vi "generate-analog-out-multiple-channels.vi"(11 "error in":errorcluster) -> (15 "error out":errorcluster)   [LabVIEW 2020]
uses:
  <vilib>/Utility/error.llb/DialogType.ctl
  <vilib>/DAQmx/write.llb/DAQmx Write (Analog 1D Wfm NChan NSamp).vi
  <vilib>/Utility/file.llb/Read Delimited Spreadsheet (string).vi
  <vilib>/DAQmx/create/channels.llb/DAQmx Create Channel (AO-Voltage-Basic).vi
  <vilib>/DAQmx/configure/timing.llb/DAQmx Timing (Use Waveform).vi
  <vilib>/DAQmx/miscellaneous.llb/DAQmx Fill In Error Info.vi
panel:
  out "Waveform Chart 4":waveform(dbl)(graph)
  out "Waveform Chart 3":waveform(dbl)(graph)
  out "number of samples written per channel":u32
  out "all rows of data":string[][](array[string])
  out "subarray":dbl[](array[numeric])
  in  "Array":dbl[][](array[numeric])
  out "Waveform Chart 2":waveform(dbl)(graph)
  out "Waveform Chart 1":waveform(dbl)(graph)
  out "Waveform Chart All":waveform(dbl)[](graph)
  in  "Delta T":dbl=0.0005
  in  "stop":bool
  in  "Physical Channel CH0":tag="DAQ1/ao0"
  in  "EMG Data File":path=path "C:/data/four-columns-of-data-by100.csv"
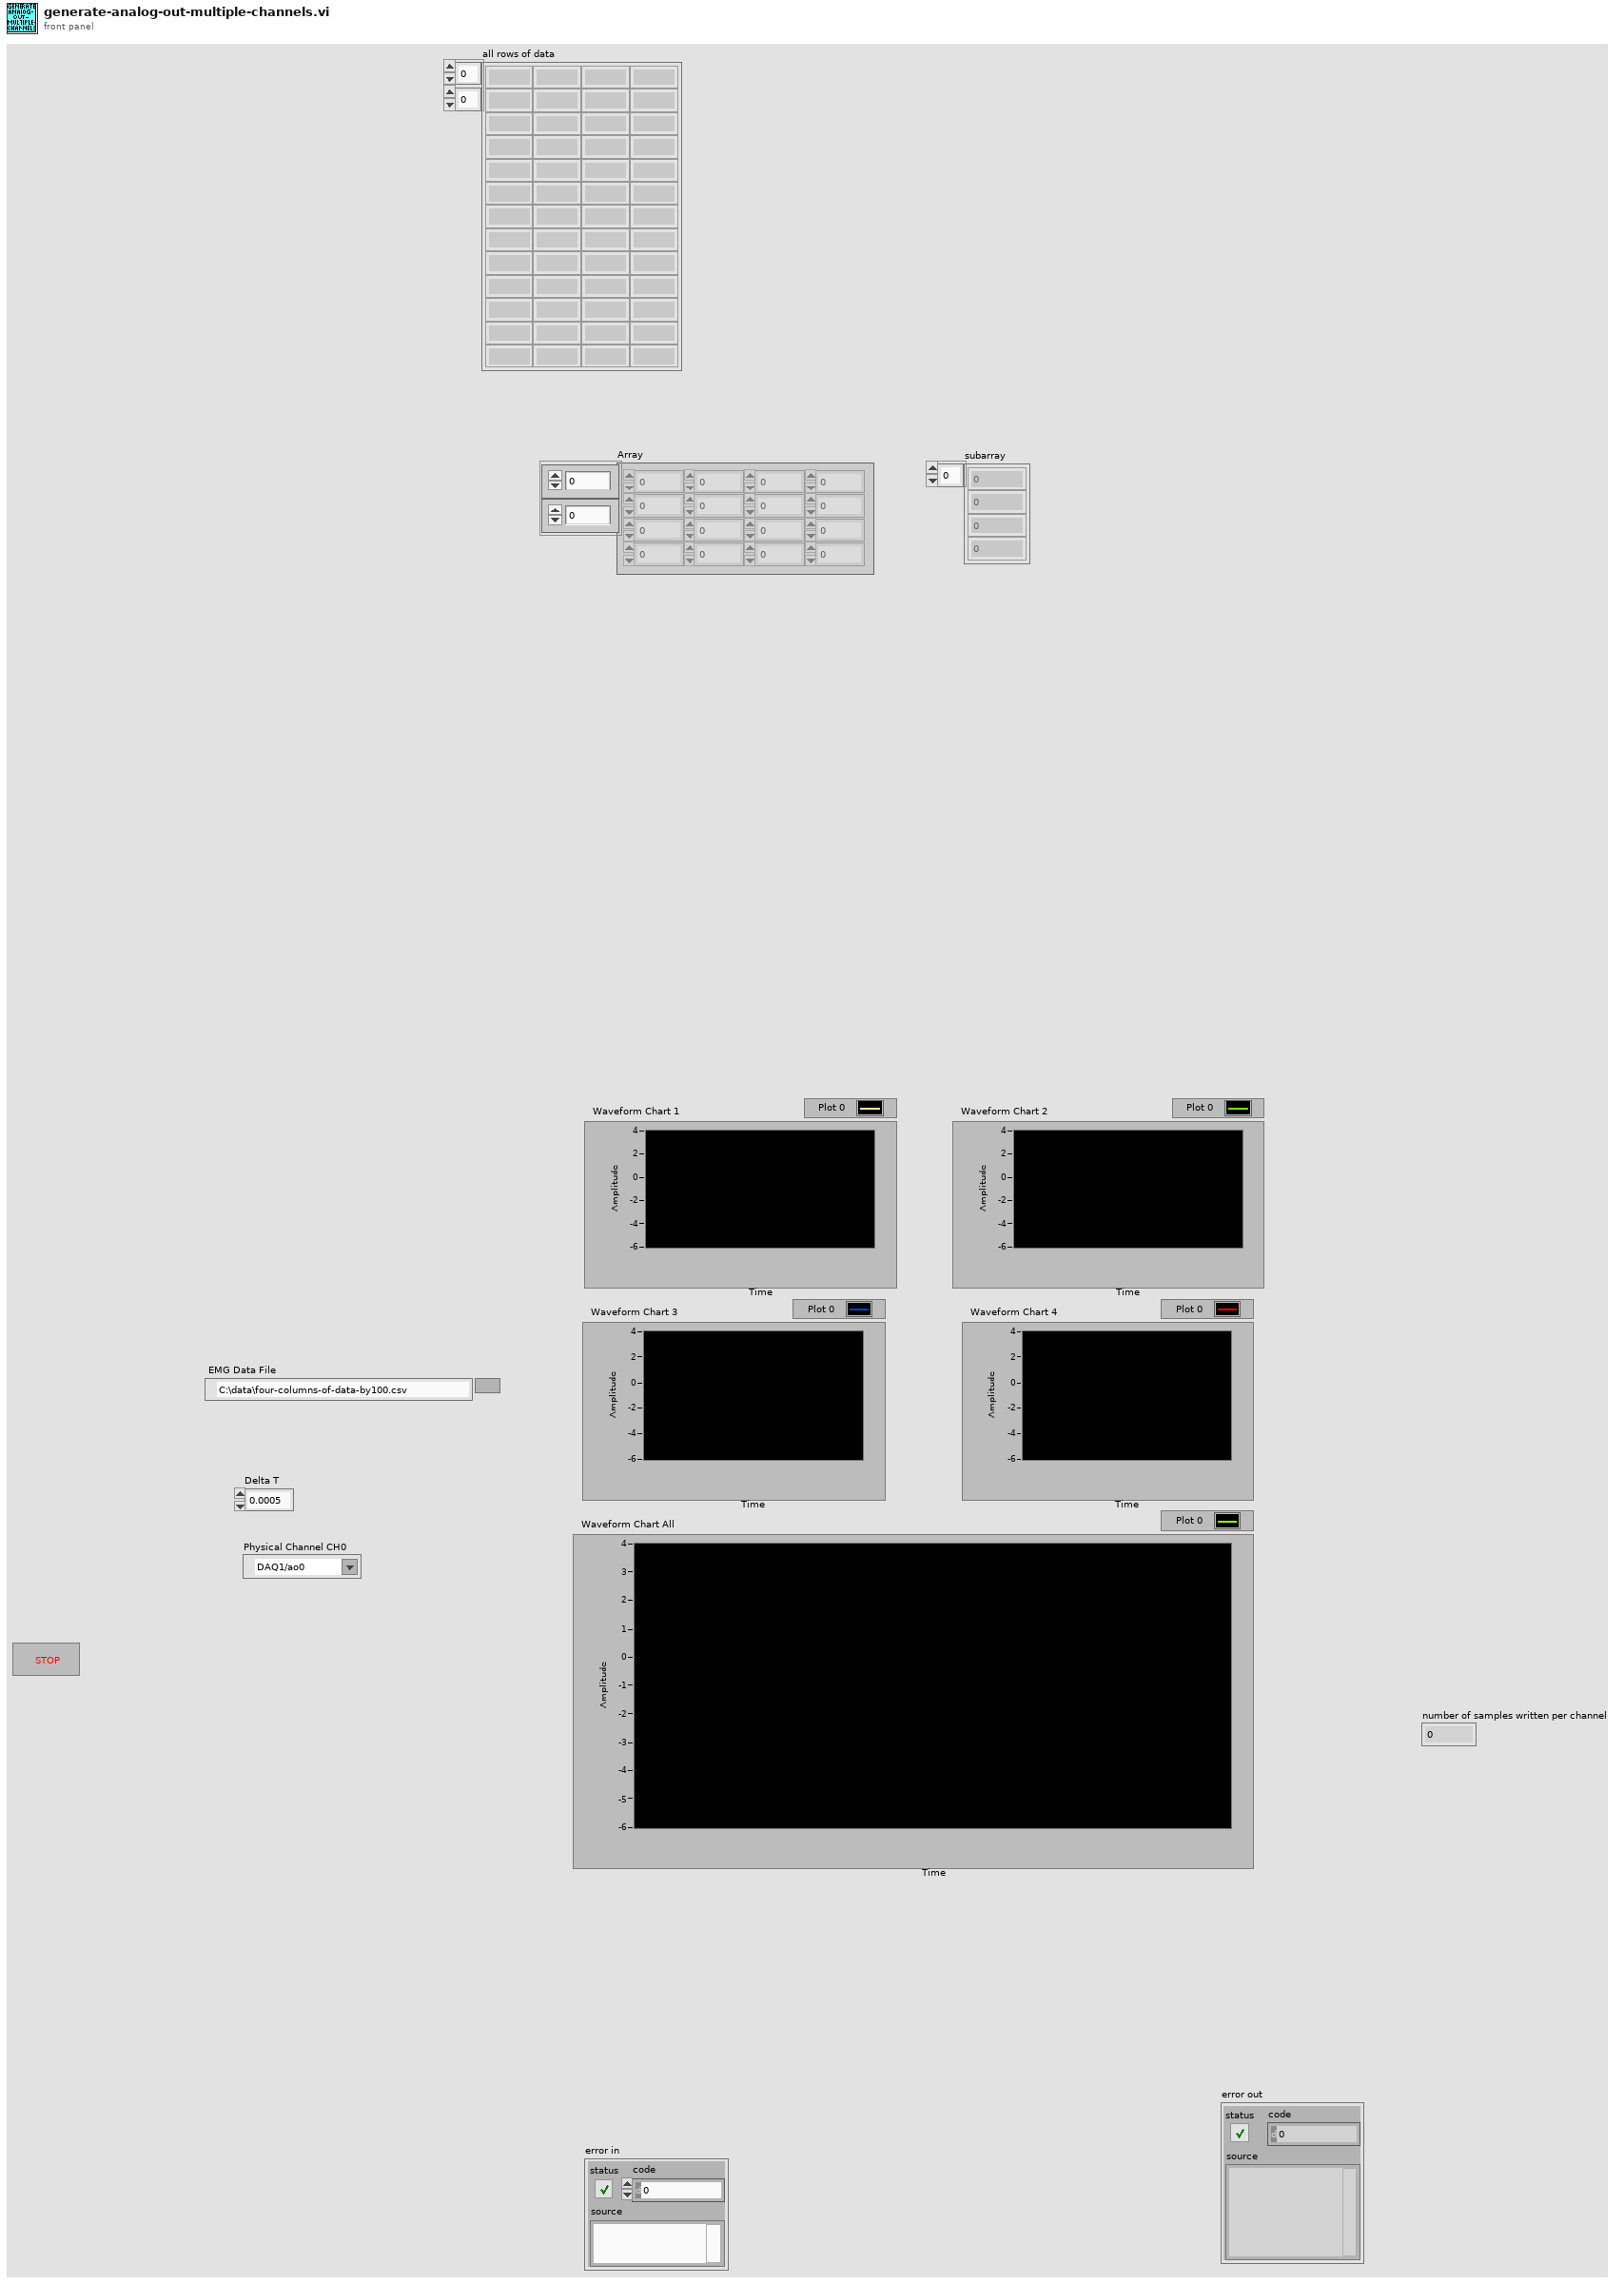
[diagram p1: front panel]
types:
  T1 = typedef "DialogType.ctl" = u16
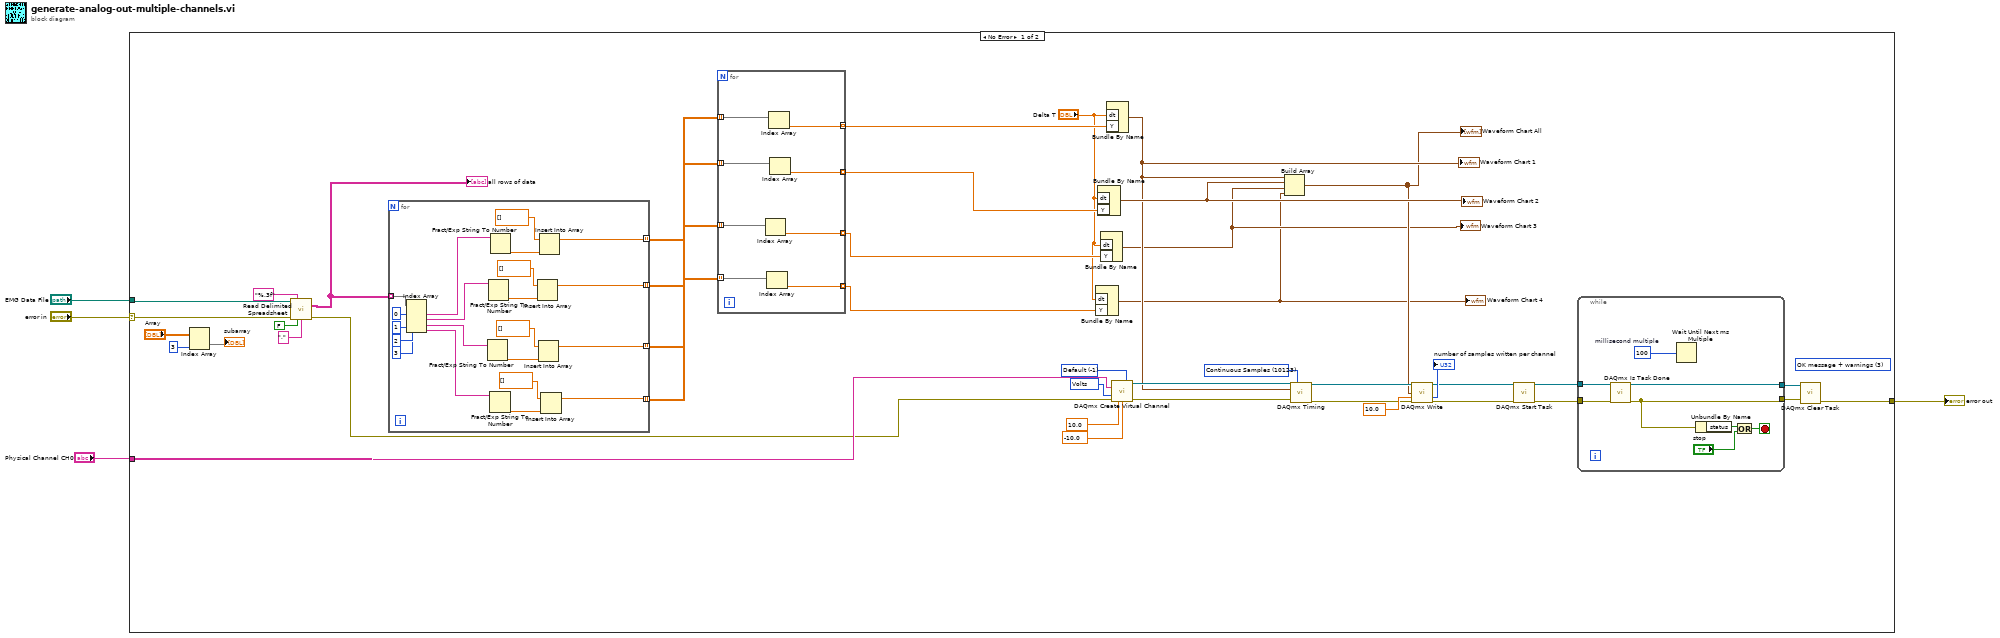
[diagram p0: block diagram]
diagram:
  n1 = case shown="No Error" "error in" {
    selector: "error in" -> [w25 w85]
    tunnel: [w7 w85] -> w3
    tunnel: "EMG Data File" -> [w29 _]
    tunnel: "Physical Channel CH0" -> [w35 _]
    frame No Error {
      w36 = 10348 items=["Volts"=10348, "From Custom Scale"=10065] ("units")
      w37 = -1 items=["Default"=-1, "RSE"=10083, "Differential"=10106, "Pseudodifferential"=12529] ("output terminal configuration")
      (unwired) T1 3 items=["no dialog", "OK message", "continue or stop message", "OK message + warnings", "continue/stop + warnings"] ("type of dialog (OK msg:1)")
      w47 = 10123 items=["Finite Samples"=10178, "Continuous Samples"=10123] ("sample mode")
      n2 = Index Array(array="Array", index (col)=3 ("disabled index (col)")) -> (element=→"subarray":dbl[])  [unwired: 1 in]
      n3 = call-poly <vilib>:"Read Delimited Spreadsheet.vi"("file path (dialog if empty)"=w29, "format (%s)"="%.3f" ("format (%.3f)"), "error in (no error)"=w25, "transpose? (F)"=FALSE, "delimiter (\\t)"="," ("delimiter (\\t)")) -> ("all rows"=w24:string[][], "error out"=w14:errorcluster)  [unwired: 5 in, 4 out]
      "all rows of data" <- w24
      n4 = for {
        tunnel: w24 -> [w76] mode=indexing
        tunnel: [w70] -> w23 mode=indexing
        tunnel: [w61] -> w21 mode=indexing
        tunnel: [w60] -> w19 mode=indexing
        tunnel: [w57] -> w18 mode=indexing
        n5 = Index Array(array=w76, index #1=0 ("index"), index #2=1 ("index"), index #3=2 ("index"), index #4=3 ("index")) -> (element #1=w68:string, element #2=w63:string, element #3=w62:string, element #4=w56:string)
        n6 = Fract/Exp String To Number(string=w62) -> (number=w65:dbl)  [unwired: 3 in, 1 out]
        n7 = Fract/Exp String To Number(string=w63) -> (number=w67:dbl)  [unwired: 3 in, 1 out]
        n8 = Fract/Exp String To Number(string=w56) -> (number=w59:dbl)  [unwired: 3 in, 1 out]
        n9 = Fract/Exp String To Number(string=w68) -> (number=w71:dbl)  [unwired: 3 in, 1 out]
        n10 = Insert Into Array(array=dbl[] [] ("Y"), new element=w67) -> (w61:dbl[])  [unwired: 1 in]
        n11 = Insert Into Array(array=dbl[] [], new element=w65) -> (w60:dbl[])  [unwired: 1 in]
        n12 = Insert Into Array(array=dbl[] [] ("Y"), new element=w71) -> (w70:dbl[])  [unwired: 1 in]
        n13 = Insert Into Array(array=dbl[] [], new element=w59) -> (w57:dbl[])  [unwired: 1 in]
      }
      n14 = for {
        tunnel: w23 -> [w55] mode=indexing
        tunnel: [w54] -> w22 mode=indexing
        tunnel: w21 -> [w53] mode=indexing
        tunnel: [w52] -> w20 mode=indexing
        tunnel: w19 -> [w51] mode=indexing
        tunnel: w18 -> [w50] mode=indexing
        tunnel: [w49] -> w10 mode=indexing
        tunnel: [w48] -> w8 mode=indexing
        n15 = Index Array(array=w51) -> (element=w49:dbl)  [unwired: 1 in]
        n16 = Index Array(array=w50) -> (element=w48:dbl)  [unwired: 1 in]
        n17 = Index Array(array=w55) -> (element=w54:dbl)  [unwired: 1 in]
        n18 = Index Array(array=w53) -> (element=w52:dbl)  [unwired: 1 in]
      }
      n19 = Bundle By Name("dt"="Delta T", "Y"=w8) -> (w5:waveform(dbl))  [unwired: 1 in]
      "Waveform Chart 4" <- w5
      n20 = Bundle By Name("dt"="Delta T", "Y"=w20) -> (w17:waveform(dbl))  [unwired: 1 in]
      "Waveform Chart 2" <- w17
      n21 = Bundle By Name("dt"="Delta T", "Y"=w10) -> (w6:waveform(dbl))  [unwired: 1 in]
      "Waveform Chart 3" <- w6
      n22 = Bundle By Name("dt"="Delta T", "Y"=w22) -> (w12:waveform(dbl))  [unwired: 1 in]
      "Waveform Chart 1" <- w12
      n23 = call-poly <vilib>:"DAQmx Create Virtual Channel.vi"("maximum value"=10.0 ("Maximum Value"), "minimum value"=-10.0 ("Minimum Value"), "output terminal configuration"=w37, "physical channels"=w35, "units"=w36, "error in"=w14) -> ("task out"=w34:refnum<k21>, "error out"=w33:errorcluster)  [unwired: 8 in]
      n24 = Build Array(w12, w17, w6, w5) -> (w11:waveform(dbl)[])
      "Waveform Chart All" <- w11
      n25 = call-poly <vilib>:"DAQmx Timing.vi"("task/channels in"=w34, "sample mode"=w47, "waveform"=w12, "error in"=w33) -> ("task out"=w16:refnum<k21>, "error out"=w40:errorcluster)  [unwired: 10 in]
      n26 = call-poly <vilib>:"DAQmx Write.vi"("task/channels in"=w16, "data"=w11, "timeout"=10.0 ("Wirite Timeout"), "error in"=w40) -> ("task out"=w13:refnum<k21>, "number of samples written per channel"=→"number of samples written per channel":u32, "error out"=w46:errorcluster)  [unwired: 9 in]
      n27 = call <vilib>:"DAQmx Start Task.vi"("task/channels in"=w13, "error in"=w46) -> ("task out"=w43:refnum<k21>, "error out"=w44:errorcluster)  [unwired: 12 in]
      n28 = while {
        tunnel: w43 -> [w84]
        tunnel: [w83] -> w42
        tunnel: w44 -> [w82]
        tunnel: [w78] -> w41
        stop <- w80 stop-if-true
        w81 = u32 100  # millisecond multiple
        n29 = call <vilib>:"DAQmx Is Task Done.vi"("task/channels in"=w84, "error in"=w82) -> ("task out"=w83:refnum<k21>, "error out"=w78:errorcluster)  [unwired: 11 in, 1 out]
        n30 = Wait Until Next ms Multiple(millisecond multiple=w81) -> ()  [unwired: 1 out]
        n31 = Unbundle By Name(w78) -> ("status"=w77:bool)
        n32 = Or(x=w77, y="stop") -> (x .or. y?=w80:bool)
      }
      n33 = call <vilib>:"DAQmx Clear Task.vi"("task in"=w42, "error in"=w41) -> ("error out"=w7:errorcluster)  [unwired: 13 in]
    }
    frame Error {
    }
  }
  "error out" <- w3
